vi "Initialize.vi"(8 "error in (no error)":errorcluster, 11 "VICI Electronic Actuator":T1) -> (0 "error out":errorcluster, 1 "Initialized":bool, 2 "No Valve Connected":bool, 3 "VICI Electronic Actuator":T1)   [LabVIEW 2018, in "VICI Electronic Actuator.lvlib"]
uses:
  D-O Module Folder/DIO Valve/VICI Electronic Actuator.lvlib
  VICI Electronic Actuator Settings.ctl
  <vilib>/Instr/_visa.llb/VISA Configure Serial Port (Instr).vi
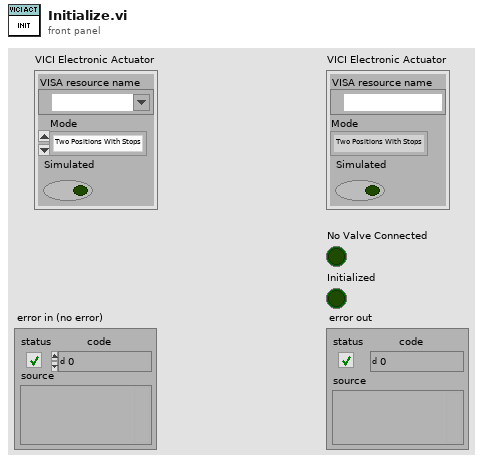
[diagram p1: front panel]
types:
  T1 = typedef "VICI Electronic Actuator.lvlib/VICI Electronic Actuator Settings.ctl" = cluster{"VISA resource name":refnum<visa-resource-name>, "Mode":enum16{"Two Positions With Stops", "Two Positions Without Stops", "Mutiposition"}, "Simulated":bool}
  T2 = enum16{"Two Positions With Stops", "Two Positions Without Stops", "Mutiposition"}
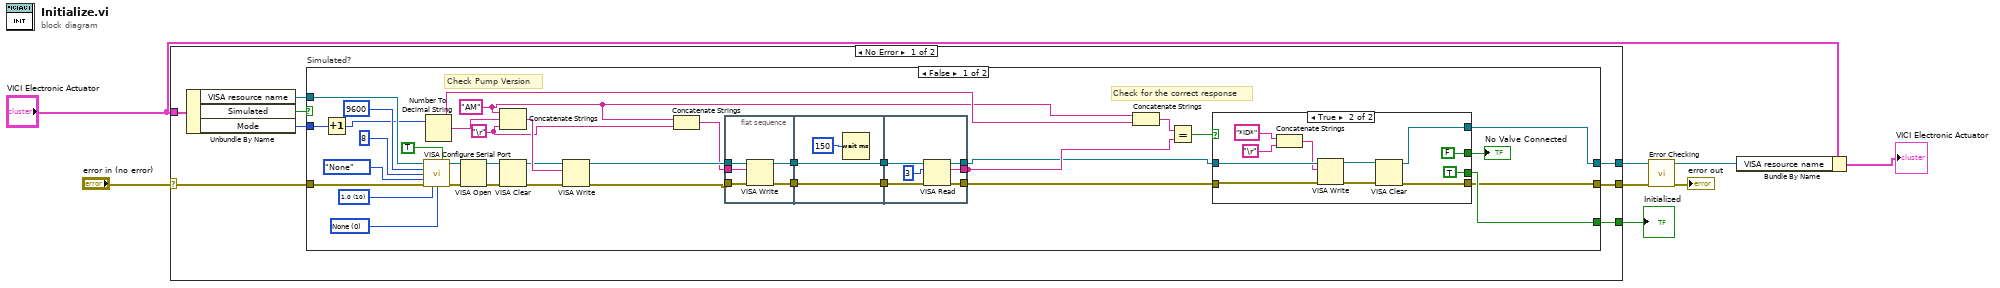
[diagram p0: block diagram]
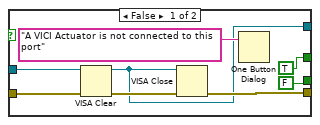
[diagram p2: hidden frame]
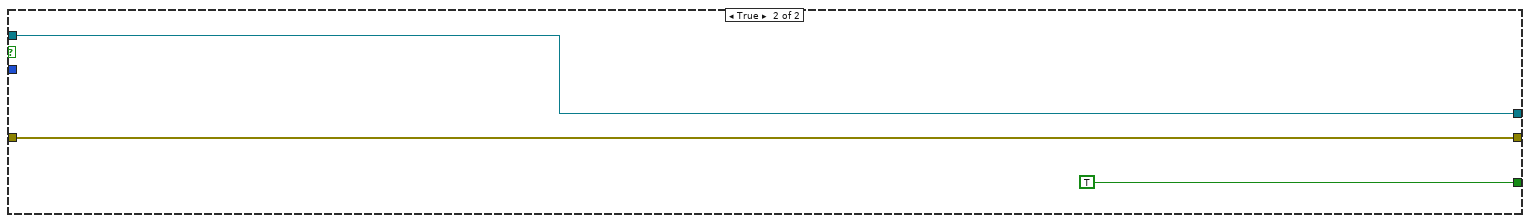
[diagram p3: hidden frame]
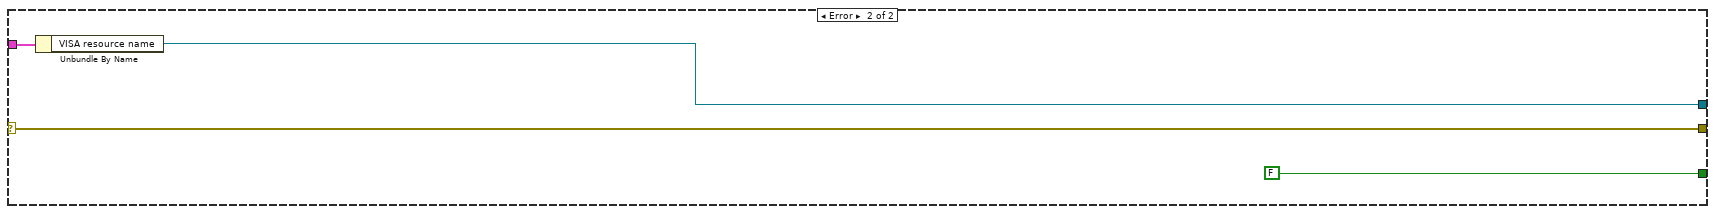
[diagram p4: hidden frame]
diagram:
  n1 = case shown="No Error" "error in (no error)" {
    selector: "error in (no error)" -> [w16 w92]
    tunnel: "VICI Electronic Actuator" -> [w13 w91]
    tunnel: [w14 w92] -> w6
    tunnel: [w11 w90] -> w7
    tunnel: [w9 FALSE] -> w3
    frame No Error {
      n2 = Unbundle By Name(w13) -> ("VISA resource name"=w12:refnum<visa-resource-name>, "Simulated"=w15:bool, "Mode"=w10:T2)
      n3 = case "Simulated?" shown="False" w15 {
        tunnel: w16 -> [w46 w88]
        tunnel: [w17 w88] -> w14
        tunnel: [w18 w87] -> w11
        tunnel: w12 -> [w44 w87]
        tunnel: w10 -> [w34 _]
        tunnel: [w35 TRUE] -> w9
        frame False {
          w23 = "AM" ("string")
          w26 = "\r"
          w48 = u16 0 items=["None", "XON/XOFF", "RTS/CTS", "XON/XOFF & RTS/CTS", "DTR/DSR", "XON/XOFF & DTR/DSR"] ("flow control (0:none)")
          w49 = u16 10 items=["1.0"=10, "1.5"=15, "2.0"=20] ("stop bits (10: 1 bit)")
          # "Check for the correct response"
          # "Check Pump Version"
          n4 = Increment(x=w34) -> (x+1=w33:T2)
          n5 = call-poly "VISA Configure Serial Port"("VISA resource name"=w44, "Enable Termination\nChar (T)"=TRUE ("Enable Termination\nChar (T)"), "baud rate (9600)"=u32 9600, "data bits (8)"=u16 8, "parity (0:none)"=enum16{"None", "Odd", "Even", "Mark", "Space"}."None", "error in (no error)"=w46, "stop bits (10: 1 bit)"=w49, "flow control (0:none)"=w48) -> ("VISA resource name out"=w45:refnum<visa-resource-name>, "error out"=w47:errorcluster)  [unwired: 6 in]
          n6 = Number To Decimal String(number=w33) -> (decimal integer string=w24:string)  [unwired: 1 in]
          n7 = VISA Open(error in (no error)=w47, VISA resource name=w45) -> (VISA resource name=w41:refnum<visa-resource-name>, error out=w38:errorcluster)  [unwired: 3 in]
          n8 = Concatenate Strings(w23, w24, w26) -> (w42:string)
          n9 = VISA Clear(VISA resource name=w41, error in (no error)=w38) -> (VISA resource name out=w40:refnum<visa-resource-name>, error out=w39:errorcluster)
          n10 = VISA Write(VISA resource name=w40, write buffer=w42, error in (no error)=w39) -> (VISA resource name out=w28:refnum<visa-resource-name>, error out=w27:errorcluster)  [unwired: 1 out]
          n11 = Concatenate Strings(w23, w26) -> (w25:string)
          n12 = flat-sequence {
            tunnel: w25 -> [w57]
            tunnel: [w56] -> w32
            tunnel: [w55] -> w31
            tunnel: w28 -> [w54]
            tunnel: w27 -> [w53]
            tunnel: [w59] -> w30
            tunnel: w32 -> [w59]
            tunnel: w31 -> [w58]
            tunnel: [w58] -> w29
            tunnel: [w66] -> w19
            tunnel: [w61] -> _
            tunnel: [w65] -> w20
            tunnel: w30 -> [w63]
            tunnel: w29 -> [w62]
            tunnel: [w61] -> w22
            frame #0 {
              n13 = VISA Write(VISA resource name=w54, write buffer=w57, error in (no error)=w53) -> (VISA resource name out=w56:refnum<visa-resource-name>, error out=w55:errorcluster)  [unwired: 1 out]
            }
            frame #1 {
              n14 = Wait (ms)(milliseconds to wait=u32 150) -> ()  [unwired: 1 out]
            }
            frame #2 {
              n15 = VISA Read(VISA resource name=w63, byte count=u32 3, error in (no error)=w62) -> (VISA resource name out=w65:refnum<visa-resource-name>, read buffer=w61:string, error out=w66:errorcluster)  [unwired: 1 out]
            }
          }
          n16 = Concatenate Strings(w23, w24) -> (w21:string)
          n17 = Equal?(x=w21, y=w22) -> (x = y?=w43:bool)
          n18 = case shown="True" w43 {
            tunnel: w20 -> [w68 w83]
            tunnel: w19 -> [w70 w82]
            tunnel: [TRUE FALSE] -> w36
            tunnel: [w72 w78] -> w17
            tunnel: [FALSE TRUE] -> w35
            tunnel: [w67 w79] -> w18
            frame False {
              n19 = VISA Clear(VISA resource name=w68, error in (no error)=w70) -> (VISA resource name out=w67:refnum<visa-resource-name>, error out=w69:errorcluster)
              n20 = VISA Close(VISA resource name=w67, error in (no error)=w69) -> (error out=w72:errorcluster)
              n21 = One Button Dialog(message="A VICI Actuator is not connected to this port") -> ()  [unwired: 1 in, 1 out]
            }
            frame True {
              n22 = Concatenate Strings("*ID*" ("string"), "\r") -> (w75:string)
              n23 = VISA Write(VISA resource name=w83, write buffer=w75, error in (no error)=w82) -> (VISA resource name out=w80:refnum<visa-resource-name>, error out=w81:errorcluster)  [unwired: 1 out]
              n24 = VISA Clear(VISA resource name=w80, error in (no error)=w81) -> (VISA resource name out=w79:refnum<visa-resource-name>, error out=w78:errorcluster)
            }
          }
          "No Valve Connected" <- w36
        }
        frame True {
        }
      }
    }
    frame Error {
      n25 = Unbundle By Name(w91) -> ("VISA resource name"=w90:refnum<visa-resource-name>)
    }
  }
  "Initialized" <- w3
  n26 = call "Error Checking.vi"("error in (no error)"=w6, "VISA resource name"=w7) -> ("error out"=→"error out":errorcluster, "VISA resource name"=w4:refnum<visa-resource-name>)  [unwired: 7 in, 1 out]
  n27 = Bundle By Name(cluster="VICI Electronic Actuator", "VISA resource name"=w4) -> (→"VICI Electronic Actuator":T1)
